vi "hardware_apply_settings.vi"(8 "error in (no error)":errorcluster, 11 "hydraharp in":refnum<class "hydraharp.lvclass">) -> (0 "error out":errorcluster, 3 "hydraharp out":refnum<class "hydraharp.lvclass">)   [LabVIEW 2015, in "hydraharp.lvclass"]
uses:
  hydraharp.lvclass
  hydraharp.lvclass/hydraharp.ctl
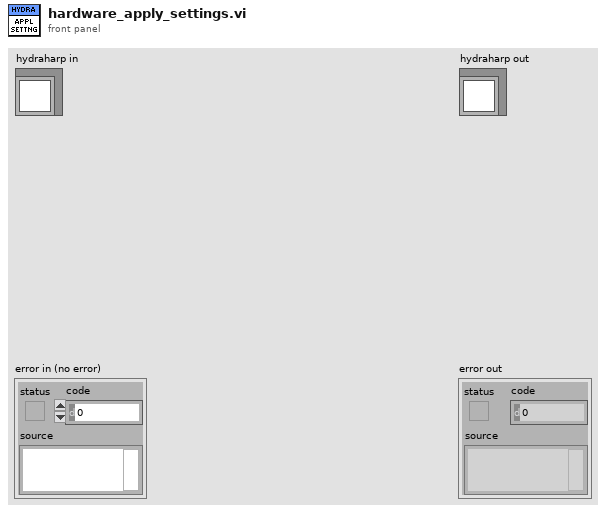
[diagram p1: front panel]
types:
  T1 = typedef "hpanel_sync_settings.ctl" = cluster{"snc_count":i32, "snc_level":i32, "snc_ZeroX":i32, "snc_offs":i32, "sync_div":T2}
  T2 = typedef "hpanel_sync_div.ctl" = enum16{"1", "2", "4", "8"}
  T3 = typedef "hpanel_channel_settings.ctl" = cluster{"ch_counts":i32, "ch_level":i32, "ch_ZeroX":i32, "ch_offs":i32}
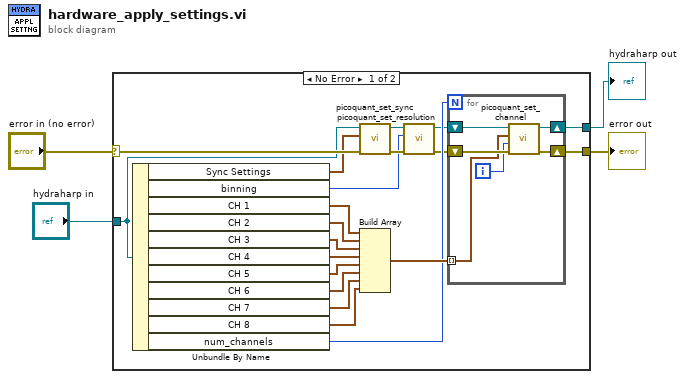
[diagram p0: block diagram]
diagram:
  n1 = case shown="No Error" "error in (no error)" {
    selector: "error in (no error)" -> [w12 w31]
    tunnel: "hydraharp in" -> [w10 w32]
    tunnel: [w23 w32] -> w2
    tunnel: [w22 w31] -> w1
    frame No Error {
      n2 = Unbundle By Name(w10) -> ("Sync Settings"=w11:T1, "binning"=w7:i32, "CH 1"=w17:T3, "CH 2"=w16:T3, "CH 3"=w15:T3, "CH 4"=w14:T3, "CH 5"=w21:T3, "CH 6"=w20:T3, "CH 7"=w19:T3, "CH 8"=w18:T3, "num_channels"=w13:i32)
      n3 = call-dynamic "picoquant_set_sync.vi"("error in (no error)"=w12, "Sync Settings"=w11, "hydraharp in"=w10) -> ("error out"=w9:errorcluster, "hydraharp out"=w8:refnum<class "hydraharp.lvclass">)  [unwired: 7 in]
      n4 = Build Array(w17, w16, w15, w14, w21, w20, w19, w18) -> (w24:T3[])
      n5 = call-dynamic "picoquant_set_resolution.vi"("error in (no error)"=w9, "resolution 2^x (ps)"=w7, "hydraharp in"=w8) -> ("error out"=w6:errorcluster, "hydraharp out"=w5:refnum<class "hydraharp.lvclass">)  [unwired: 7 in]
      n6 = for {
        N: w13 -> [_]
        shift-right: [w28] -> w23
        shift-left: w5 -> [w27]
        tunnel: w24 -> [w25] mode=indexing
        shift-right: [w29] -> w22
        shift-left: w6 -> [w30]
        i -> [w26]
        n7 = call-dynamic "picoquant_set_channel.vi"("error in (no error)"=w30, "channel_num"=w26, "ch_settings"=w25, "hydraharp in"=w27) -> ("error out"=w29:errorcluster, "hydraharp out"=w28:refnum<class "hydraharp.lvclass">)  [unwired: 6 in]
      }
    }
    frame Error {
    }
  }
  "error out" <- w1
  "hydraharp out" <- w2
